vi "限幅滤波.vi"() -> ()   [LabVIEW 2018]
panel:
  out "限幅滤波值":dbl
  in  "限幅值":i32
  in  "实时采样值":i32
  in  "停止":bool
  in  "采样数":i32
  out "字符串":string="限幅滤波"
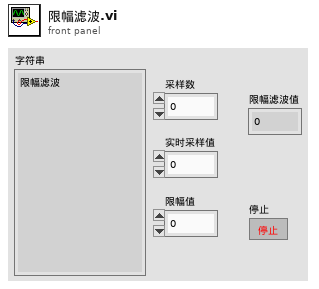
[diagram p1: front panel]
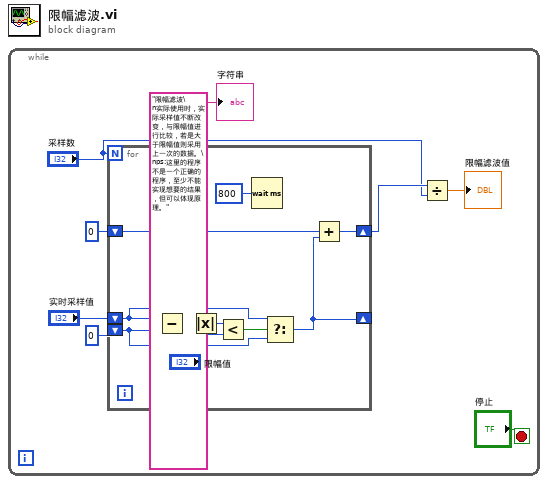
[diagram p0: block diagram]
diagram:
  n1 = while {
    stop <- "停止" stop-if-true
    n2 = for {
      N: "采样数" -> [_]
      shift-right: [w10] -> w5
      shift-left: 0 -> [w11]
      shift-right: [w12] -> _
      shift-left: "实时采样值" -> [w14]
      shift-left: 0 ("实时采样值") -> [w13]
      n3 = Subtract(x=w14, y=w13) -> (x-y=w18:i32)
      n4 = Absolute Value(x=w18) -> (abs(x)=w17:i32)
      n5 = Less?(x=w17, y="限幅值") -> (x < y?=w15:bool)
      n6 = Wait (ms)(milliseconds to wait=u32 800 ("等待时间（毫秒）")) -> ()  [unwired: 1 out]
      n7 = Select(t=w14, s=w15, f=w13) -> (s? t:f=w12:i32)
      n8 = Add(x=w11, y=w12) -> (x+y=w10:i32)
    }
    n9 = Divide(x=w5, y="采样数") -> (x/y=→"限幅滤波值":dbl)
    "字符串" <- "限幅滤波\n实际使用时，实际采样值不断改变，与限幅值进行比较，若是大于限幅值则采用上一次的数据。\nps:这里的程序不是一个正确的程序，至少不能实现想要的结果，但可以体现原理。"
  }
